vi "Set Trigger Mode.vi"(8 "error in (no error)":errorcluster, 10 "Trigger Mode":T1, 11 "PXIe5105 in":refnum<class "PXIe5105.lvclass">) -> (0 "error out":errorcluster, 3 "PXIe5105 out":refnum<class "PXIe5105.lvclass">)   [LabVIEW 2018, in "PXIe5105.lvlib" / "PXIe5105.lvclass"]
doc: "This Override sets the trigger to Auto or Normal mode. Auto generates a trigger even if one has not been detected after certain perios of time. Normal waits for trigger detection."
uses:
  PXIe5105.lvclass
  PPLs/Oscilloscope/Parent/Oscilloscope.lvlibp/Custom Controls/Trigger Mode.ctl
  PPLs/Oscilloscope/Parent/Oscilloscope.lvlibp
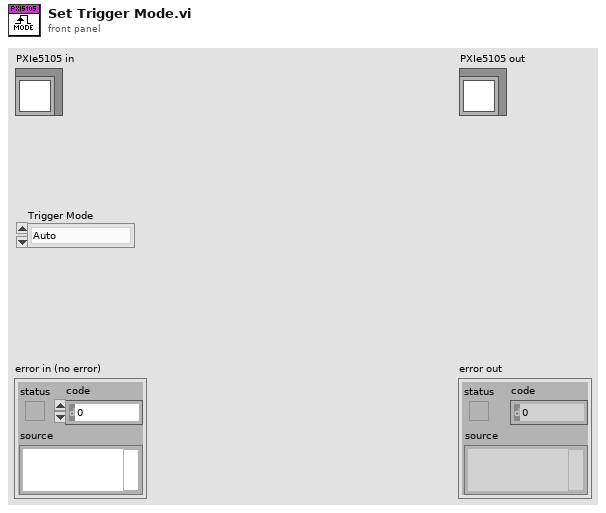
[diagram p1: front panel]
types:
  T1 = typedef "Oscilloscope.lvlibp/Trigger Mode.ctl" = enum16{"Auto", "Normal"}
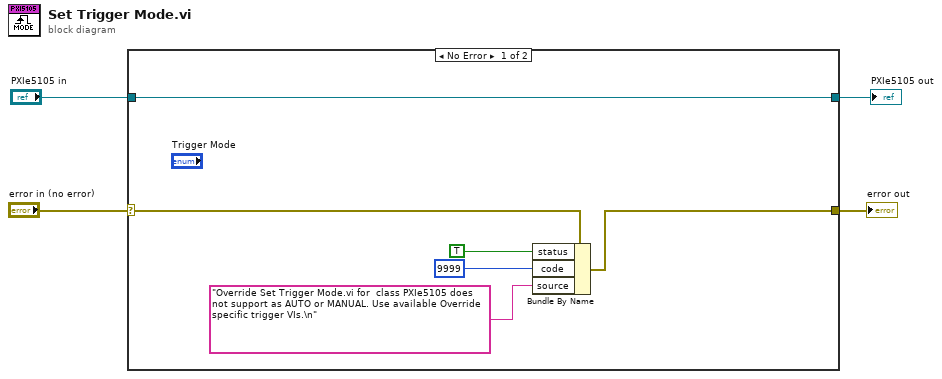
[diagram p0: block diagram]
diagram:
  n1 = case shown="No Error" "error in (no error)" {
    selector: "error in (no error)" -> [w7 w12]
    tunnel: [w6 w12] -> w3
    tunnel: [w5 w11] -> w2
    tunnel: "PXIe5105 in" -> [w5 w11]
    frame No Error {
      n2 = Bundle By Name(cluster=w7, "status"=TRUE, "code"=9999, "source"="Override Set Trigger Mode.vi for  class PXIe5105 does not support as AUTO or MANUAL. Use available Override specific trigger VIs.\n") -> (w6:errorcluster)
    }
    frame Error {
    }
  }
  "error out" <- w3
  "PXIe5105 out" <- w2
